vi "LVObject to JSON - Enable LabVIEW Extensions - Is Passed to Serializable Class.vi"() -> ()   [LabVIEW 2017, in "JSON Serializable Serializer Tests.lvlib"]
uses:
  JSON Serializable Serializer Tests.lvlib
  JSON Serializable Serializer/JSON Serializable Serializer.lvclass
  Mock JSON Serializable/Mock JSON Serializable.lvclass/Mock JSON Serializable.ctl
  <vilib>/addons/_JKI Toolkits/Caraya/classes/Assert/Assert False.vi
  <vilib>/addons/_JKI Toolkits/Caraya/classes/Test/Test.lvclass
  <vilib>/addons/_JKI Toolkits/Caraya/classes/Assert/Assert.lvclass
  Mock JSON Serializable/Mock JSON Serializable.lvclass
panel:
  out "error out":errorcluster
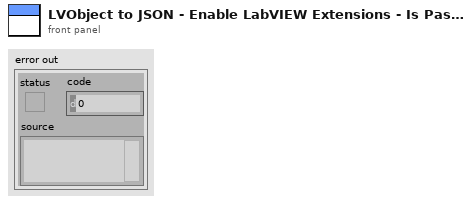
[diagram p1: front panel]
types:
  T1 = cluster{"LVClass Serializer":refnum<class "JSONtext LVClass Serializer.lvclass">, "enable LabVIEW extensions? (T)":bool, "Pretty Print?":bool, "error in (no error)":errorcluster}
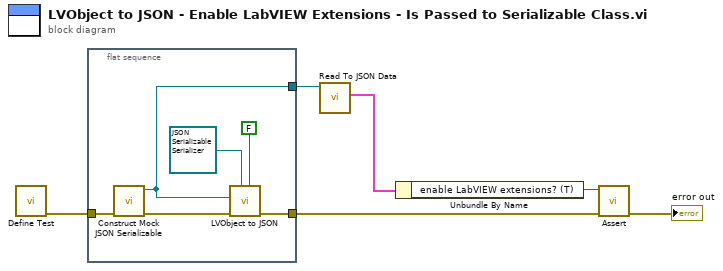
[diagram p0: block diagram]
diagram:
  n1 = call <vilib>:"Define Test.vi"() -> ("error out"=w5:errorcluster)  [unwired: 11 in]
  n2 = flat-sequence {
    tunnel: [w10] -> w6
    tunnel: w5 -> [w11]
    tunnel: [w8] -> w2
    frame #0 {
      n3 = call "Construct Mock JSON Serializable.vi"("error in (no error)"=w11) -> ("error out"=w9:errorcluster, "Mock JSON Serializable"=w8:refnum<class "Mock JSON Serializable.lvclass">)  [unwired: 9 in]
      n4 = call-dynamic "LVObject to JSON.vi"("enable LabVIEW extensions? (T)"=FALSE, "JSON Serializer in"=refnum<class "JSON Serializable Serializer.lvclass"> refnum ("JSON Serializer.lvclass"), "error in (no error)"=w9, "Object"=w8) -> ("error out"=w10:errorcluster)  [unwired: 6 in, 1 out]
    }
  }
  n5 = call "Read To JSON Data.vi"("Mock JSON Serializable in"=w2) -> ("To JSON Data"=w1:T1)  [unwired: 9 in, 1 out]
  n6 = Unbundle By Name(w1) -> ("enable LabVIEW extensions? (T)"=w3:bool)
  n7 = call-poly <vilib>:"Assert.vi"("error in (no error)"=w6, "False?"=w3) -> ("error out"=→"error out":errorcluster)  [unwired: 9 in]
